vi "format floats[] for database.vi"(4 "Numbers":dbl[](array[numeric])) -> (1 "Insertion Strings":string[](array[string]))   [LabVIEW 2022 SP3, in "hse-db-ado.lvlib" / "ADO-DB-Driver.lvlib"]
doc: "Format array of float for database (either engineering format or NULL)\n\n____\nHAMPEL SOFTWARE ENGINEERING v1.4.0 (2023-12-19 09:52)"
uses:
  ADO-DB-Driver.lvlib
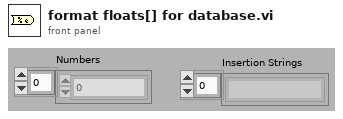
[diagram p1: front panel]
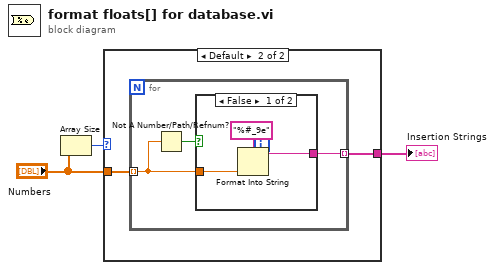
[diagram p0: block diagram]
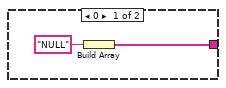
[diagram p2: hidden frame]
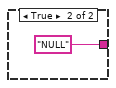
[diagram p3: hidden frame]
diagram:
  n1 = Array Size(array="Numbers") -> (size(s)=w3:i32)
  n2 = case shown="Default" w3 {
    tunnel: "Numbers" -> [_ w6]
    tunnel: [w4 w7] -> w1
    frame 0 {
      n3 = Build Array("NULL") -> (w4:string[])
    }
    frame Default {
      n4 = for {
        tunnel: [w10] -> w7 mode=indexing
        tunnel: w6 -> [w8] mode=indexing
        n5 = Not A Number/Path/Refnum?(number/path/refnum=w8) -> (NaN/Path/Refnum?=w9:bool)
        n6 = case shown="False" w9 {
          tunnel: [w11 "NULL"] -> w10
          tunnel: w8 -> [w12 _]
          frame False {
            n7 = Format Into String(format string="%#_9e", w12) -> (resulting string=w11:string)  [unwired: 2 in, 1 out]
          }
          frame True {
          }
        }
      }
    }
  }
  "Insertion Strings" <- w1
